vi "End Receive Data.vi"(0 "Tovey9150 in":refnum<class "Tovey 9150.lvclass">, 11 "error in (no error)":errorcluster) -> (4 "Tovey9150 out":refnum<class "Tovey 9150.lvclass">, 6 "Data Present":bool, 8 "A":dbl, 10 "B":dbl, 15 "error out":errorcluster)   [LabVIEW 2015, in "Tovey 9150.lvclass"]
uses:
  Tovey 9150.lvclass
  Tovey 9150.lvclass/Tovey 9150.ctl
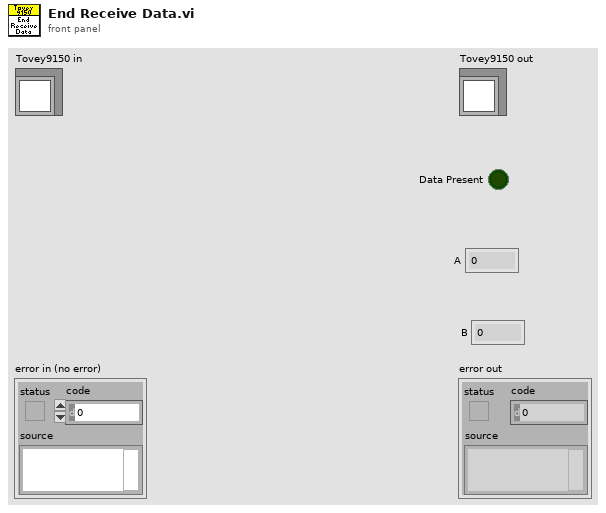
[diagram p1: front panel]
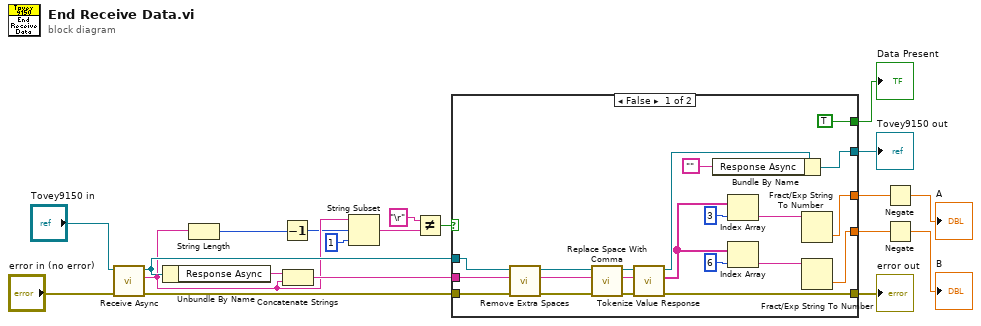
[diagram p0: block diagram]
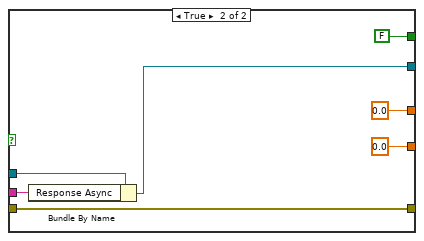
[diagram p2: hidden frame]
diagram:
  n1 = call "Receive Async.vi"("error in (no error)"="error in (no error)", "Tovey9150 in"="Tovey9150 in") -> ("error out"=w15:errorcluster, "Response"=w8:string, "Tovey9150 out"=w16:refnum<class "Tovey 9150.lvclass">)  [unwired: 7 in]
  n2 = Unbundle By Name(w16) -> ("Response Async"=w18:string)
  n3 = String Length(string=w8) -> (length=w11:i32)
  n4 = Decrement(x=w11) -> (x-1=w7:i32)
  n5 = Concatenate Strings(w18, w8) -> (w17:string)
  n6 = String Subset(string=w8, offset (0)=w7, length (rest)=1 ("length (rest)")) -> (substring=w6:string)
  n7 = Not Equal?(x="\r", y=w6) -> (x != y?=w9:bool)
  n8 = case shown="False" w9 {
    tunnel: w17 -> [w38 w44]
    tunnel: w16 -> [w41 w45]
    tunnel: w15 -> [w35 w42]
    tunnel: [w32 w42] -> w13
    tunnel: [w26 0.0] -> w2
    tunnel: [w25 0.0] -> w4
    tunnel: [TRUE FALSE] -> w14
    tunnel: [w21 w43] -> w12
    frame False {
      n9 = call "Remove Extra Spaces.vi"("error in (no error)"=w35, "Input"=w38, "Tovey 9150 in"=w41) -> ("error out"=w34:errorcluster, "Output"=w37:string, "Tovey 9150 out"=w40:refnum<class "Tovey 9150.lvclass">)  [unwired: 6 in]
      n10 = call "Replace Space With Comma.vi"("error in (no error)"=w34, "Input"=w37, "Tovey 9150 in"=w40) -> ("error out"=w33:errorcluster, "Output"=w36:string, "Tovey 9150 out"=w39:refnum<class "Tovey 9150.lvclass">)  [unwired: 6 in]
      n11 = call "Tokenize Value Response.vi"("error in (no error)"=w33, "Input"=w36, "Tovey 9150 in"=w39) -> ("error out"=w32:errorcluster, "Tokens"=w29:string[], "Tovey 9150 out"=w23:refnum<class "Tovey 9150.lvclass">)  [unwired: 6 in]
      n12 = Bundle By Name(cluster=w23, "Response Async"="") -> (w21:refnum<class "Tovey 9150.lvclass">)
      n13 = Index Array(array=w29, index=3) -> (element=w27:string)
      n14 = Index Array(array=w29, index=6) -> (element=w28:string)
      n15 = Fract/Exp String To Number(string=w27) -> (number=w26:dbl)  [unwired: 3 in, 1 out]
      n16 = Fract/Exp String To Number(string=w28) -> (number=w25:dbl)  [unwired: 3 in, 1 out]
    }
    frame True {
      n17 = Bundle By Name(cluster=w45, "Response Async"=w44) -> (w43:refnum<class "Tovey 9150.lvclass">)
    }
  }
  "error out" <- w13
  "Tovey9150 out" <- w12
  "Data Present" <- w14
  n18 = Negate(x=w2) -> (-x=→"A":dbl)
  n19 = Negate(x=w4) -> (-x=→"B":dbl)
